vi "Read PacketFormatter.vi"(11 "DebuggingTerminal in":refnum<class "DebuggingTerminal.lvclass">) -> (2 "PacketFormatter":refnum<class "PacketFormatter.lvclass">, 3 "DebuggingTerminal out":refnum<class "DebuggingTerminal.lvclass">)   [LabVIEW 2013, in "MQTT Base.lvlib" / "DebuggingTerminal.lvclass"]
uses:
  DebuggingTerminal.lvclass
  PacketFormatter/PacketFormatter.lvclass
  DebuggingTerminal.lvclass/DebuggingTerminal.ctl
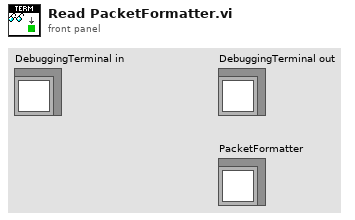
[diagram p1: front panel]
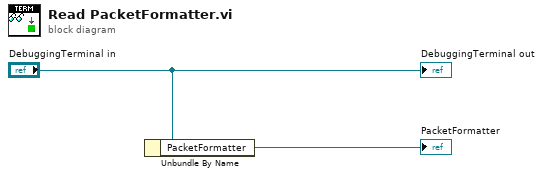
[diagram p0: block diagram]
diagram:
  n1 = Unbundle By Name("DebuggingTerminal in") -> ("PacketFormatter"=→"PacketFormatter":refnum<class "PacketFormatter.lvclass">)
  "DebuggingTerminal out" <- "DebuggingTerminal in"
